vi "Rio_Coordinate_Array (DONE).vi"(7 "Coordinate Selection":bool, 8 "Error In":errorcluster, 9 "Home Position":dbl[](array[numeric]), 10 "Coordinate":dbl[](array[numeric])) -> (0 "Error Out":errorcluster, 2 "Y":dbl, 3 "X":dbl)   [LabVIEW 2017]
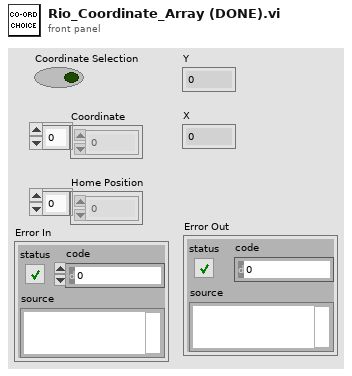
[diagram p1: front panel]
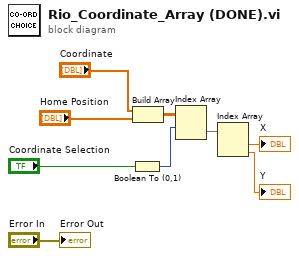
[diagram p0: block diagram]
diagram:
  n1 = Boolean To (0,1)(Boolean="Coordinate Selection") -> (0, 1=w9:i16)
  n2 = Build Array("Coordinate", "Home Position") -> (w4:dbl[][])
  n3 = Index Array(array=w4, index (row)=w9) -> (element=w5:dbl[])  [unwired: 1 in]
  n4 = Index Array(array=w5) -> (element #1=→"X":dbl, element #2=→"Y":dbl)  [unwired: 2 in]
  "Error Out" <- "Error In"
